vi "Table-Prevent non-numerics in first X columns.vi"(6 "Filter this number of first columns":i32=3, 8 "error in (no error)":errorcluster, 9 "New Value in":string[][](array[string]), 11 "Old Value in":string[][](array[string])) -> (0 "error out":errorcluster, 2 "Filtered array":string[][](array[string]), 3 "Discard":bool)   [LabVIEW 2020]
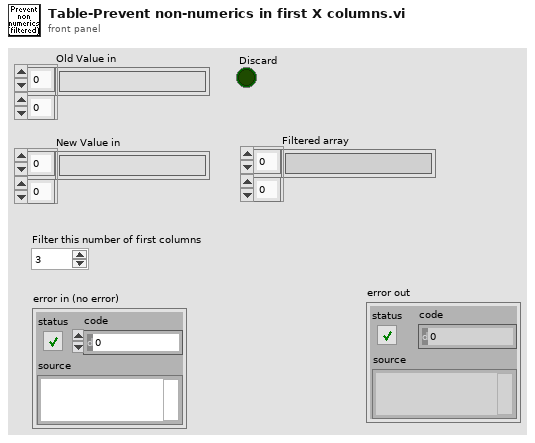
[diagram p1: front panel]
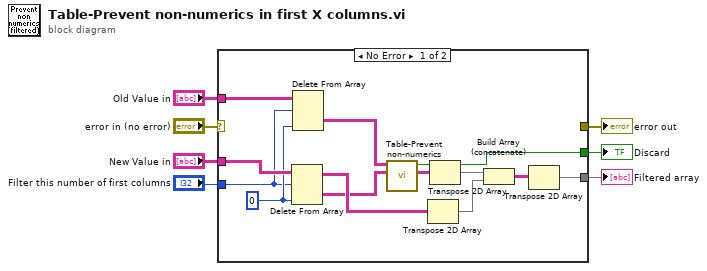
[diagram p0: block diagram]
diagram:
  n1 = case shown="No Error" "error in (no error)" {
    selector: "error in (no error)" -> [_ w22]
    tunnel: [w19 w21] -> w7
    tunnel: "New Value in" -> [w12 w21]
    tunnel: [w11 _] -> w5
    tunnel: "Old Value in" -> [w9 _]
    tunnel: [_ w22] -> w2
    tunnel: "Filter this number of first columns" -> [w8 _]
    frame No Error {
      w10 = 0 ("disabled index (col)")
      n2 = Delete From Array(array=w12, length=w8, index (col)=w10) -> (deleted portion=w13:string[][], array with subset deleted=w16:string[][])  [unwired: 1 in]
      n3 = Delete From Array(array=w9, length=w8, index (col)=w10) -> (deleted portion=w20:string[][])  [unwired: 1 in, 1 out]
      n4 = call <userlib>:"Table-Prevent non-numerics.vi"("NewVal in"=w13, "OldVal"=w20) -> ("Val out"=w14:string[][], "Discard"=w11:bool)  [unwired: 7 in, 1 out]
      n5 = Transpose 2D Array(2D array=w16) -> (transposed array=w18:string[][])
      n6 = Transpose 2D Array(2D array=w14) -> (transposed array=w17:string[][])
      n7 = Build Array (concatenate)(w17, w18) -> (w15:string[][])
      n8 = Transpose 2D Array(2D array=w15) -> (transposed array=w19:string[][])
    }
    frame Error {
    }
  }
  "Filtered array" <- w7
  "Discard" <- w5
  "error out" <- w2
